vi "Create.vi"(8 "error in (no error)":errorcluster) -> (0 "error out":errorcluster, 3 "State out":refnum<class "State.lvclass">)   [LabVIEW 2017, in "Promise Future.lvlib" / "State.lvclass"]
uses:
  State.lvclass
  State Core.ctl
  State.lvclass/State.ctl
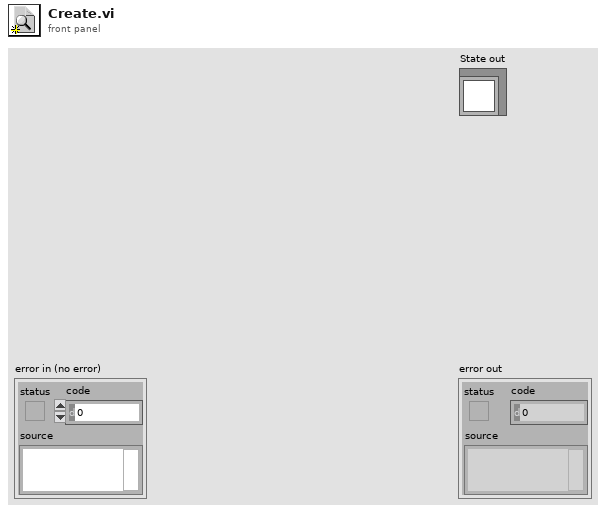
[diagram p1: front panel]
types:
  T1 = typedef "Promise Future.lvlib/State.lvclass/State Core.ctl" = cluster{"Value":refnum<queue>, "Callbacks":refnum<queue>, "Semaphore":T2}
  T2 = typedef "Semaphore RefNum" = refnum<k1>
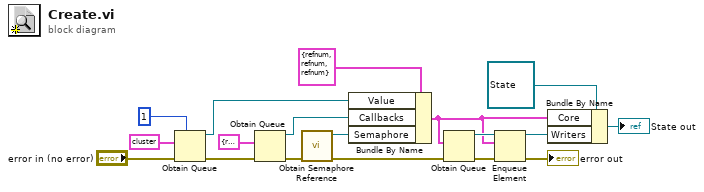
[diagram p0: block diagram]
diagram:
  n1 = Obtain Queue(max queue size (-1, unlimited)=1, element data type=cluster{"Value":variant, "Error":errorcluster} {"Value"=variant, "Error"={"status"=FALSE, "code"=0, "source"=""}} ("output cluster"), error in (no error)="error in (no error)") -> (queue out=w13:refnum<queue>, error out=w11:errorcluster)  [unwired: 2 in, 1 out]
  n2 = Obtain Queue(element data type=cluster{"Callback":refnum<vi>, "Scope":variant} {"Callback"=refnum, "Scope"=variant} ("output cluster"), error in (no error)=w11) -> (queue out=w7:refnum<queue>, error out=w12:errorcluster)  [unwired: 3 in, 1 out]
  n3 = call <vilib>:"Obtain Semaphore Reference.vi"("error in (no error)"=w12) -> ("error out"=w5:errorcluster, "semaphore"=w8:T2)  [unwired: 4 in, 1 out]
  n4 = Bundle By Name(cluster=T1 {"Value"=refnum, "Callbacks"=refnum, "Semaphore"=refnum} ("Cluster"), "Value"=w13, "Callbacks"=w7, "Semaphore"=w8) -> (w3:T1)
  n5 = Obtain Queue(element data type=w3, error in (no error)=w5) -> (queue out=w4:refnum<queue>, error out=w6:errorcluster)  [unwired: 3 in, 1 out]
  n6 = Enqueue Element(queue=w4, element=w3, error in (no error)=w6) -> (queue out=w2:refnum<queue>, error out=→"error out":errorcluster)  [unwired: 1 in, 1 out]
  n7 = Bundle By Name(cluster=refnum<class "State.lvclass"> refnum ("State out"), "Core"=w3, "Writers"=w2) -> (→"State out":refnum<class "State.lvclass">)
